vi "Add Ephemeral Peel.vi"(9 "BananaPeel":refnum<class "BananaPeel.lvclass">, 11 "Banana":refnum<class "Banana.lvclass">) -> (3 "Banana":refnum<class "Banana.lvclass">)   [LabVIEW 2021, in "Bananas.lvlib" / "Platano.lvclass"]
uses:
  Platano/Platano.lvclass
  Banana.lvclass
  BananaPeel/BananaPeel.lvclass
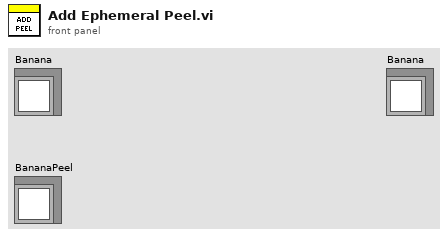
[diagram p1: front panel]
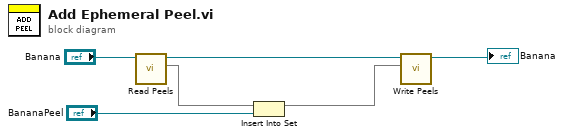
[diagram p0: block diagram]
diagram:
  n1 = call "Read Peels.vi"("Banana in"="Banana") -> ("Peels"=w2:set{refnum<class "BananaPeel.lvclass">}, "Banana out"=w3:refnum<class "Banana.lvclass">)  [unwired: 8 in, 1 out]
  n2 = Insert Into Set(10:"BananaPeel", 11:w2) -> (3:w1:set{refnum<class "BananaPeel.lvclass">})  [unwired: 1 out]
  n3 = call "Write Peels.vi"("Peels"=w1, "Banana in"=w3) -> ("Banana out"=→"Banana":refnum<class "Banana.lvclass">)  [unwired: 8 in, 1 out]
